vi "tester.vi"() -> ()   [LabVIEW 2013]
uses:
  <vilib>/Platform/TimedLoop/XDataNode/timing_clust.ctl
  <vilib>/Platform/TimedLoop/XDataNode/nitl_modes.ctl
  <vilib>/Platform/TimedLoop/XDataNode/wakeup.ctl
  <vilib>/rvi/Emulation/niFpgaSctlEmulationGetInTimedLoop.vi
  <vilib>/rvi/DataTransferAndStorage/Container/Common/niFpgaContainerGetUniqueNameForEmu.vi
  <vilib>/rvi/DataTransferAndStorage/Container/Common/niFpgaContainerSetEmuInfo.vi
  <vilib>/rvi/eio/common/nirviEmuReportErrorAndStop.vi
  <vilib>/rvi/Emulation/niFpgaEmulationReportErrorSimple.vi
  <vilib>/rvi/Emulation/niFpgaGetClockAttributes.vi
  <vilib>/rvi/Emulation/niFpgaCriticalErrorInLSC.vi
  <vilib>/rvi/DataTransferAndStorage/Container/Common/niFpgaContainerExecOnDevCompGetState.vi
  <vilib>/rvi/DataTransferAndStorage/Register/Emulation/niFpgaRegisterEmulationFpgaImpl.vi
  <instcachedir>/0/niFpgaRegisterEmulationFpgaImpl_DCF4BC0110594B98B44A971D60CEEC4D.lvgen/niFpgaRegisterEmulationFpgaImpl_DCF4BC0110594B98B44A971D60CEEC4D_000.vi
  <vilib>/rvi/eio/common/nirviEmuTemplateMethod_errors.vi
  <vilib>/rvi/FIFO/Fifo_Resource/nirvififoEmulationWriteFpgaImpl.vi
  <vilib>/rvi/FIFO/Fifo_Resource/nirvififoEmulationReadFpgaImpl.vi
  <vilib>/Platform/TimedLoop/XDataNode/XDataNode.xnode
  <vilib>/rvi/LocalResourceManager/LocalResourceManager.xnode
  <vilib>/rvi/DataTransferAndStorage/Container/XNode/niFpgaContainer.xnode
  <vilib>/rvi/DataTransferAndStorage/Register/Emulation/niFpgaRegisterEmulationRefIn.vi
  <vilib>/eio/EIONode/EIONode.xnode
  <vilib>/rvi/FIFO/Fifo_Resource/nirvififoEmulationWrite.vi
  <vilib>/rvi/FIFO/Fifo_Resource/nirvififoEmulationRead.vi
  <vilib>/Platform/TimedLoop/XDataNode/XDNodeRunTimeDep.lvlib
panel:
  in  "Pacer":i16
  in  "PulseUpClck":u16=3
  in  "PulseWaitClck":u16=40
  out "SimOut":i16
  in  "Devider":u8=3
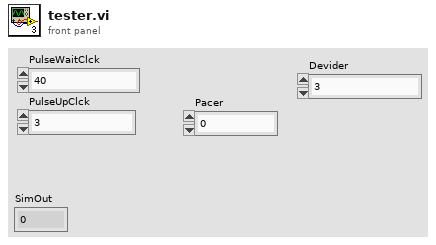
[diagram p1: front panel]
types:
  T1 = typedef "XDNodeRunTimeDep.lvlib/timing_clust.ctl" = cluster{"Expected End [f-1]":u64, "Actual End [f-1]":u64, "Finished Late? [f-1]":bool, "Expected End [i-1]":u64, "Actual End [i-1]":u64, "Finished Late? [i-1]":bool, "Expected Start [i]":u64, "Actual Start [i]":u64, "Expected Start [f]":u64, "Actual Start [f]":u64, "Source Name":string, "Structure Name":string, "Period":i64, "Deadline":i64, "Offset":i64, "Start":i64, "Priority":i32, "Timeout":i32, "Mode":T2, "Wakeup Reason":T3, "Error":errorcluster, "Source Type":string, "Secondary Source Type":string, "Global End Time":u64, "Global Start Time":u64, "Frame Duration":u64, "Iteration Duration":u64, "Assigned CPU":i32, "I/O Scan Engine Mode":u32}
  T2 = typedef "XDNodeRunTimeDep.lvlib/nitl_modes.ctl" = enum32{"No Change", "Process missed periods, maintain original phase", "Discard missed periods, maintain original phase", "Process missed periods, ignore original phase", "Discard missed periods, ignore original phase"}
  T3 = typedef "XDNodeRunTimeDep.lvlib/wakeup.ctl" = enum32{"Normal", "Aborted", "Asynchronous wakeup", "Timing source error", "Timed loop error", "Timeout"}
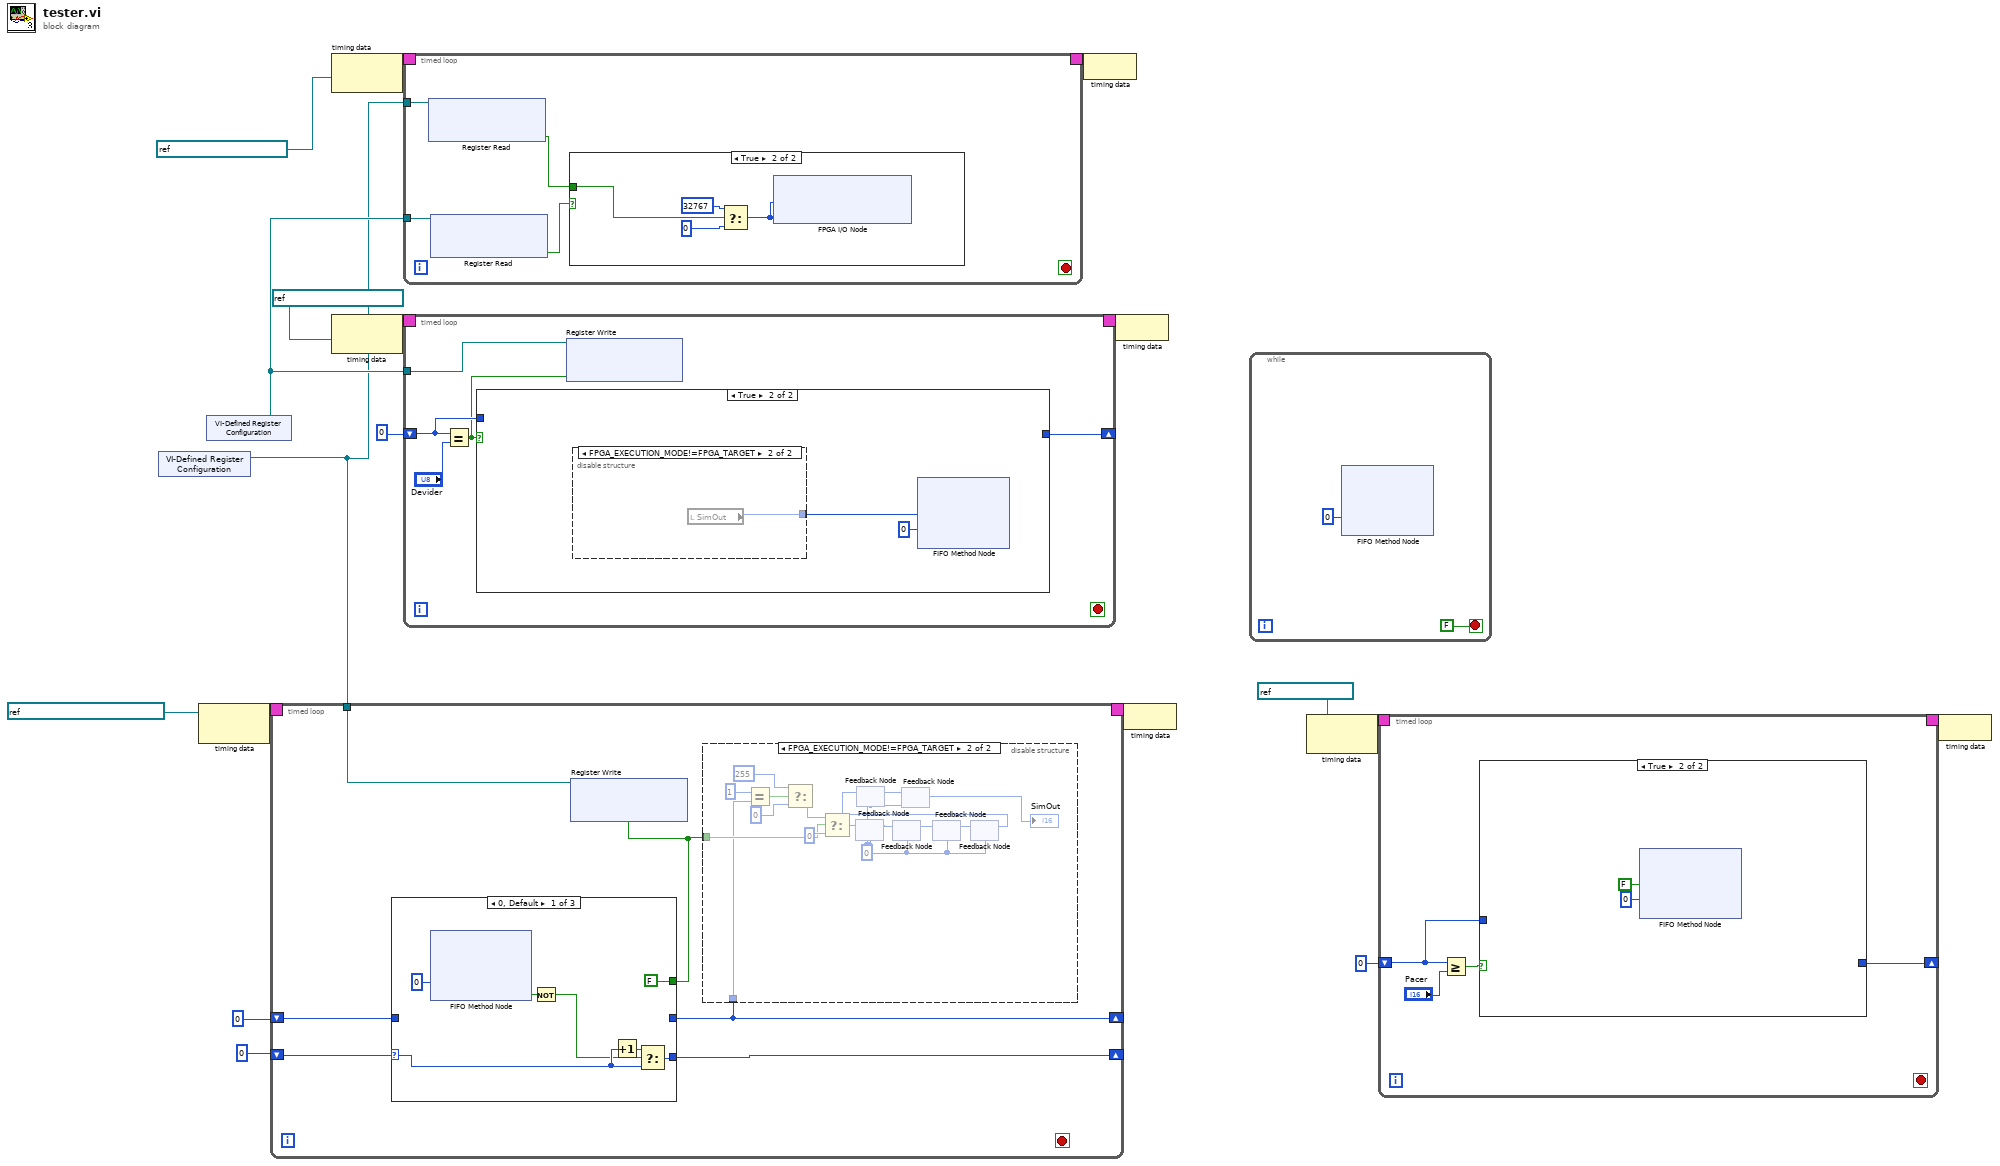
[diagram p0: block diagram]
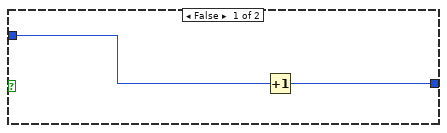
[diagram p2: hidden frame]
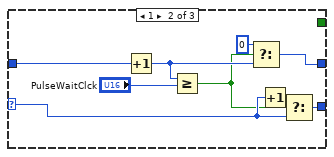
[diagram p4: hidden frame]
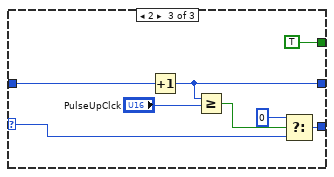
[diagram p5: hidden frame]
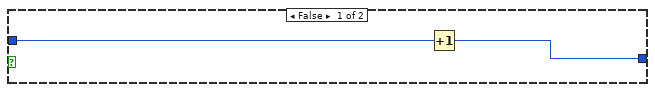
[diagram p7: hidden frame]
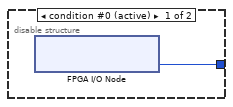
[diagram p8: hidden frame]
diagram:
  n1 = xnode ("VI-Defined Register Configuration")() -> ("Register Out"=w1:refnum<k21>)
  n2 = node-c288(refnum<k21> "IO Module\\Data Clock Div 2" ("Source Name")) -> (w11:T1)
  n3 = xnode ("VI-Defined Register Configuration")() -> ("Register Out"=w2:refnum<k21>)
  n4 = timed-loop {
    timing: w11 -> [_]
    timing-out: [_] -> w10
    shift-right: [w23] -> _
    shift-left: i16 0 -> [w24]
    shift-right: [w21] -> _
    shift-left: u16 0 -> [w22]
    tunnel: w1 -> [w20]
    stop <- _ stop-if-true
    n5 = case shown="0, Default" w24 {
      selector: w24 -> [w46 w53 w59]
      tunnel: [w47 w54 w60] -> w23
      tunnel: w22 -> [_ w56 w64]
      tunnel: [_ w50 w63] -> w21
      tunnel: [FALSE _ TRUE] -> w19
      frame 0, Default {
        n6 = xnode ("FIFO Method Node")("Timeout"=0) -> ("Timed Out?"=w43:bool)  [unwired: 1 in, 2 out]
        n7 = Not(x=w43) -> (.not. x?=w41:bool)
        n8 = Increment(x=w46) -> (x+1=w45:i16)
        n9 = Select(t=w45, s=w41, f=w46) -> (s? t:f=w47:i16)
      }
      frame 1 {
        n10 = Increment(x=w56) -> (x+1=w51:u16)
        n11 = Greater Or Equal?(x=w51, y="PulseWaitClck") -> (x >= y?=w48:bool)
        n12 = Select(t=u16 0, s=w48, f=w51) -> (s? t:f=w50:u16)
        n13 = Increment(x=w53) -> (x+1=w52:i16)
        n14 = Select(t=w52, s=w48, f=w53) -> (s? t:f=w54:i16)
      }
      frame 2 {
        n15 = Increment(x=w64) -> (x+1=w63:u16)
        n16 = Greater Or Equal?(x=w63, y="PulseUpClck") -> (x >= y?=w61:bool)
        n17 = Select(t=i16 0, s=w61, f=w59) -> (s? t:f=w60:i16)
      }
    }
    n18 = xnode ("Register Write")("Data"=w19, "Register In"=w20) -> ()  [unwired: 1 out]
    n19 = disable-structure shown="FPGA_EXECUTION_MODE!=FPGA_TARGET" {
      disable-tunnel: w19 -> [_ w32]
      disable-tunnel: w21 -> [_ w31]
      frame condition #0 (active) {
      }
      frame condition #1 {
        w35 = i16 0 ("IO Module\\AO 0")
        n20 = Equal?(x=u16 1, y=w31) -> (x = y?=w29:bool)
        n21 = Select(t=i16 255 ("IO Module\\AO 0"), s=w29, f=i16 0) -> (s? t:f=w30:i16)
        n22 = Select(t=w30, s=w32, f=i16 0 ("IO Module\\AO 0")) -> (s? t:f=w33:i16)
        n23 = feedback-in #1(w33) -> ()
        n24 = feedback #1(w35) -> (w40:i16)
        n25 = feedback #2(w35) -> (w36:i16)
        n26 = feedback #3(w35) -> (w39:i16)
        n27 = feedback-in #3(w40) -> ()
        n28 = feedback #4(w35) -> (→"SimOut":i16)
        n29 = feedback-in #4(w36) -> ()
        n30 = feedback #5(w35) -> (w38:i16)
        n31 = feedback-in #5(w39) -> ()
        n32 = feedback #6(w35) -> (w37:i16)
        n33 = feedback-in #2(w37) -> ()
        n34 = feedback-in #6(w38) -> ()
      }
    }
  }
  n35 = node-c288(refnum<k21> "IO Module\\Data Clock" ("Source Name")) -> (w16:T1)
  n36 = node-c288(refnum<k21> "IO Module\\Data Clock" ("Source Name")) -> (w18:T1)
  n37 = timed-loop {
    timing: w16 -> [_]
    timing-out: [_] -> w15
    tunnel: w2 -> [w70]
    tunnel: w1 -> [w68]
    stop <- _ stop-if-true
    n38 = xnode ("Register Read")("Register In"=w68) -> ("Data"=w67:bool)  [unwired: 1 out]
    n39 = xnode ("Register Read")("Register In"=w70) -> ("Data"=w69:bool)  [unwired: 1 out]
    n40 = case shown="True" w69 {
      tunnel: w67 -> [_ w71]
      frame False {
      }
      frame True {
        n41 = Select(t=i16 32767 ("IO Module\\AO 0"), s=w71, f=i16 0 ("IO Module\\AO 0")) -> (s? t:f=w72:i16)
        n42 = xnode "FPGA I/O Node"("IO Module\\AO 0 N-1"=w72, "IO Module\\AO 0 N"=w72) -> ()  [unwired: 2 in, 2 out]
      }
    }
  }
  n43 = timed-loop {
    timing: w18 -> [_]
    timing-out: [_] -> w17
    shift-right: [w79] -> _
    shift-left: u8 0 -> [w80]
    tunnel: w2 -> [w78]
    stop <- _ stop-if-true
    n44 = Equal?(x=w80, y="Devider") -> (x = y?=w77:bool)
    n45 = case shown="True" w77 {
      tunnel: w80 -> [w83 _]
      tunnel: [w82 _] -> w79
      frame False {
        n46 = Increment(x=w83) -> (x+1=w82:u8)
      }
      frame True {
        n47 = disable-structure shown="FPGA_EXECUTION_MODE!=FPGA_TARGET" {
          disable-tunnel: [w86 w87] -> w84
          frame condition #0 (active) {
            n48 = xnode "FPGA I/O Node"() -> ("IO Module\\AI 0"=w86:i16)  [unwired: 1 in, 1 out]
          }
          frame condition #1 {
            n49 = local read "SimOut"() -> (w87:i16)
          }
        }
        n50 = xnode ("FIFO Method Node")("Element"=w84, "Timeout"=0) -> ()  [unwired: 1 in, 2 out]
      }
    }
    n51 = xnode ("Register Write")("Data"=w77, "Register In"=w78) -> ()  [unwired: 1 out]
  }
  n52 = node-c288(w15) -> ()
  n53 = node-c288(w17) -> ()
  n54 = node-c288(w10) -> ()
  n55 = while {
    stop <- FALSE stop-if-true
    n56 = xnode ("FIFO Method Node")("Timeout"=0) -> ()  [unwired: 1 in, 3 out]
  }
  n57 = node-c288(refnum<k21> "100 MHz Clock" ("Source Name")) -> (w6:T1)
  n58 = timed-loop {
    timing: w6 -> [_]
    timing-out: [_] -> w5
    shift-right: [w93] -> _
    shift-left: i16 0 -> [w92]
    stop <- _ stop-if-true
    n59 = Greater Or Equal?(x=w92, y="Pacer") -> (x >= y?=w94:bool)
    n60 = case shown="True" w94 {
      tunnel: [w96 _] -> w93
      tunnel: w92 -> [w97 _]
      frame False {
        n61 = Increment(x=w97) -> (x+1=w96:i16)
      }
      frame True {
        n62 = xnode ("FIFO Method Node")("Element"=FALSE, "Timeout"=0) -> ()  [unwired: 1 in, 2 out]
      }
    }
  }
  n63 = node-c288(w5) -> ()
